vi "Get string lines to array.vi"(6 "Key data":string, 8 "error in (no error)":errorcluster, 9 "Key must be at start of line?":bool, 10 "Only lines with XXX?":bool, 11 "String with lines":string) -> (0 "error out":errorcluster, 2 "Lines":i32, 3 "Matching lines":string[](array[string]))   [LabVIEW 2013]
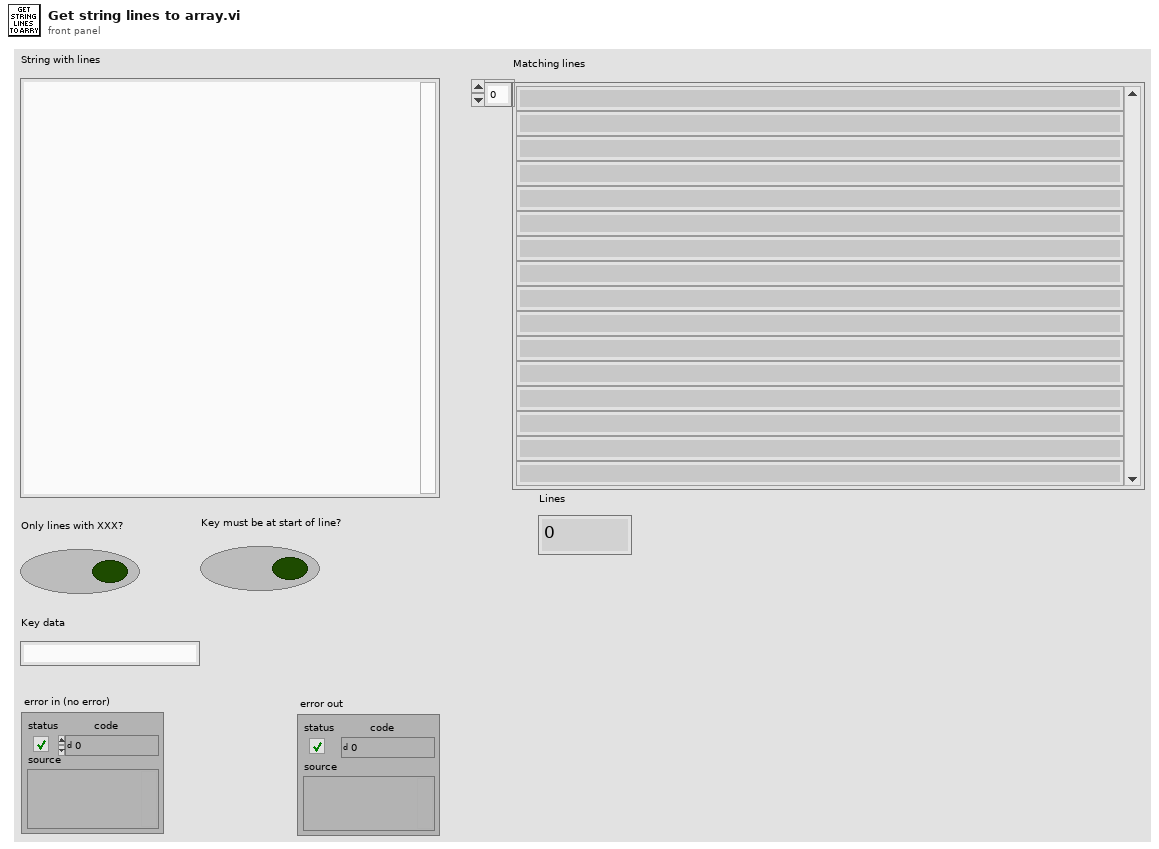
[diagram p1: front panel]
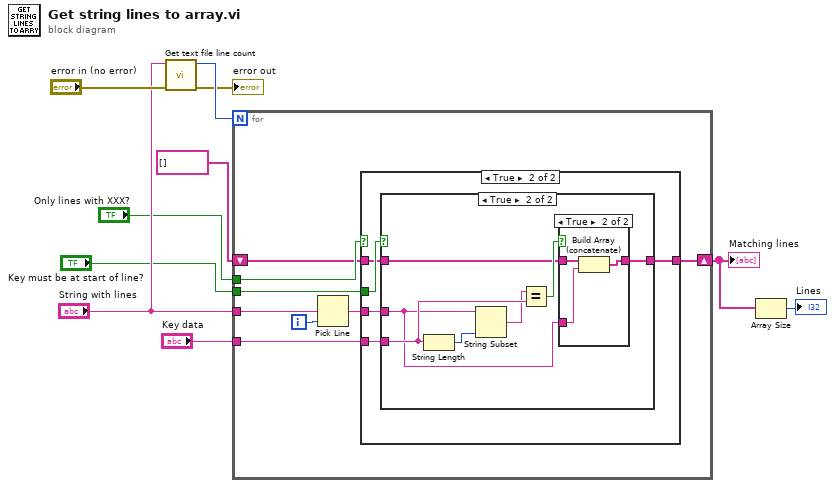
[diagram p0: block diagram]
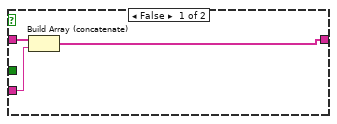
[diagram p2: hidden frame]
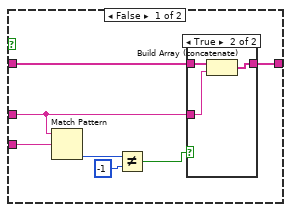
[diagram p3: hidden frame]
diagram:
  n1 = call "Get text file line count.vi"("error in (no error)"="error in (no error)", "text string"="String with lines") -> ("error out"=→"error out":errorcluster, "Line cnt"=w10:i32)  [unwired: 8 in]
  n2 = for {
    N: w10 -> [_]
    tunnel: "String with lines" -> [w18]
    tunnel: "Only lines with XXX?" -> [w16]
    tunnel: "Key must be at start of line?" -> [w15]
    tunnel: "Key data" -> [w13]
    shift-right: [w11] -> w2
    shift-left: string[] [] -> [w12]
    i -> [w17]
    n3 = Pick Line(multi-line string=w18, line index=w17) -> (output string=w14:string)  [unwired: 1 in]
    n4 = case shown="True" w16 {
      tunnel: w15 -> [_ w26]
      tunnel: w14 -> [w20 w25]
      tunnel: w13 -> [_ w24]
      tunnel: w12 -> [w21 w23]
      tunnel: [w19 w22] -> w11
      frame False {
        n5 = Build Array (concatenate)(w21, w20) -> (w19:string[])
      }
      frame True {
        n6 = case shown="True" w26 {
          tunnel: w25 -> [w28 w38]
          tunnel: w24 -> [w33 w43]
          tunnel: w23 -> [w29 w41]
          tunnel: [w27 w39] -> w22
          frame False {
            n7 = Match Pattern(string=w28, regular expression=w33) -> (offset past match=w32:i32)  [unwired: 1 in, 3 out]
            n8 = Not Equal?(x=w32, y=-1) -> (x != y?=w30:bool)
            n9 = case shown="True" w30 {
              tunnel: [w34 w37] -> w27
              tunnel: w29 -> [w34 w36]
              tunnel: w28 -> [_ w35]
              frame False {
              }
              frame True {
                n10 = Build Array (concatenate)(w36, w35) -> (w37:string[])
              }
            }
          }
          frame True {
            n11 = String Length(string=w43) -> (length=w44:i32)
            n12 = String Subset(string=w38, length (rest)=w44) -> (substring=w40:string)  [unwired: 1 in]
            n13 = Equal?(x=w40, y=w43) -> (x = y?=w42:bool)
            n14 = case shown="True" w42 {
              tunnel: w41 -> [w45 w48]
              tunnel: w38 -> [_ w47]
              tunnel: [w45 w46] -> w39
              frame False {
              }
              frame True {
                n15 = Build Array (concatenate)(w48, w47) -> (w46:string[])
              }
            }
          }
        }
      }
    }
  }
  "Matching lines" <- w2
  n16 = Array Size(array=w2) -> (size(s)=→"Lines":i32)
